vi "DEMO Motion Communication.vi"() -> ()   [LabVIEW 2018, in "MotionComm.lvclass"]
uses:
  MotionComm.lvclass
  Support/MessageQue/MessageQue.lvlib
panel:
  in  "milliseconds to wait before motion ack":u32=2000
  in  "Timeout, s on Postion Command":dbl=5.0 format="%#_13g"
  out "error out":errorcluster
  # "When wait > Timeout\nthere should be an error >>"
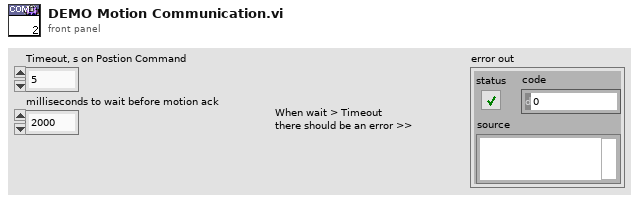
[diagram p1: front panel]
types:
  T1 = typedef "MessageQue.lvlib/MessageQue.ctl" = refnum<queue>
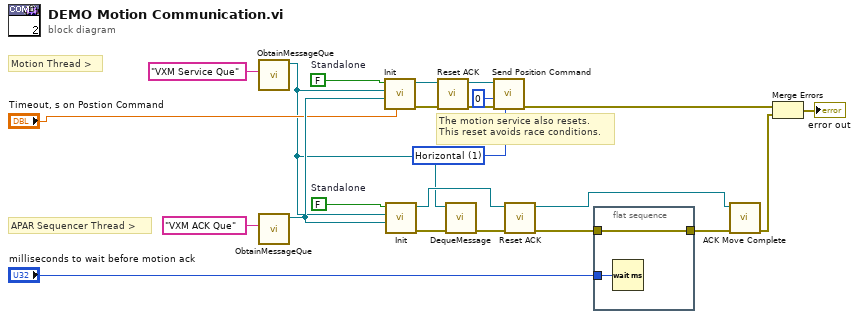
[diagram p0: block diagram]
diagram:
  w1 = u16 1 items=["Vertical", "Horizontal"] ("Polarization")
  w17 = FALSE  # Standalone
  w18 = FALSE  # Standalone
  # "The motion service also resets.\nThis reset avoids race conditions."
  # "APAR Sequencer Thread >"
  # "Motion Thread >"
  n1 = call "ObtainMessageQue.vi"("Name"="VXM Service Que") -> ("message que out"=w8:T1)  [unwired: 7 in, 3 out]
  n2 = call "ObtainMessageQue.vi"("Name"="VXM ACK Que") -> ("message que out"=w21:T1)  [unwired: 7 in, 3 out]
  n3 = call "Init.vi"("Timeout, s"="Timeout, s on Postion Command", "VXM ACK que"=w21, "VXM Svc que"=w8, "Standalone"=w17) -> ("error out"=w6:errorcluster, "MotionComm out"=w5:refnum<class "MotionComm.lvclass">)  [unwired: 6 in]
  n4 = call "Init.vi"("VXM ACK que"=w21, "VXM Svc que"=w8, "Standalone"=w18) -> ("error out"=w10:errorcluster, "MotionComm out"=w9:refnum<class "MotionComm.lvclass">)  [unwired: 7 in]
  n5 = call "Reset ACK.vi"("error in (no error)"=w6, "MotionComm in"=w5) -> ("error out"=w3:errorcluster, "MotionComm out"=w4:refnum<class "MotionComm.lvclass">)  [unwired: 8 in]
  n6 = call "DequeMessage.vi"("error in"=w10, "Message que"=w8) -> ("error out"=w7:errorcluster)  [unwired: 4 in, 5 out]
  n7 = call "Send Position Command.vi"("Polarization"=w1, "error in (no error)"=w3, "TR Module/Raster num"=0, "MotionComm in"=w4) -> ("error out"=w11:errorcluster)  [unwired: 6 in, 1 out]
  n8 = call "Reset ACK.vi"("error in (no error)"=w7, "MotionComm in"=w9) -> ("error out"=w12:errorcluster, "MotionComm out"=w13:refnum<class "MotionComm.lvclass">)  [unwired: 8 in]
  n9 = flat-sequence {
    tunnel: [w25] -> w19
    tunnel: w12 -> [w25]
    tunnel: "milliseconds to wait before motion ack" -> [w24]
    frame #0 {
      n10 = Wait (ms)(milliseconds to wait=w24) -> ()  [unwired: 1 out]
    }
  }
  n11 = call "ACK Move Complete.vi"("error in (no error)"=w19, "MotionComm in"=w13) -> ("error out"=w16:errorcluster)  [unwired: 8 in, 1 out]
  n12 = Merge Errors(w11, w16) -> (→"error out":errorcluster)
